vi "checkStatesBallPlacementEnemyTactic.vi"(9 "ballPosition(x,y)":dbl[](array[numeric]), 10 "Robot":refnum<class "Robot.lvclass">, 11 "Game in":refnum<class "Game.lvclass">) -> (1 "projectionOfQInBallPlacementLine":dbl[](array[numeric]) format="%#_13g", 2 "distance":dbl, 3 "isRobotIntereringInBallPlacement?":bool)   [LabVIEW 2021, in "BallPlacementEnemyTactic.lvclass"]
uses:
  BallPlacementEnemyTactic.lvclass
  Robot_class/Robot.lvclass
  D:/RoboIme/horie/SSL_AI/Object_class/Object.lvclass
  Game_class/Game.lvclass
  Object_class/Object.lvclass/Object.ctl
  Game_class/Game.lvclass/Game.ctl
  <vilib>/Analysis/baseanly.llb/Unit Vector (DBL).vi
  Game_class/Read Referee.vi
  Game_class/Read BallRef.vi
  Game_class/Read NewParameters.vi
  Object_class/Read x.vi
  Object_class/Read y.vi
  Referee_class/Referee.lvclass
  Ball_class/Ball.lvclass
  Utilities_class/Utilities.lvclass
  <vilib>/Analysis/NI_AALBase.lvlib
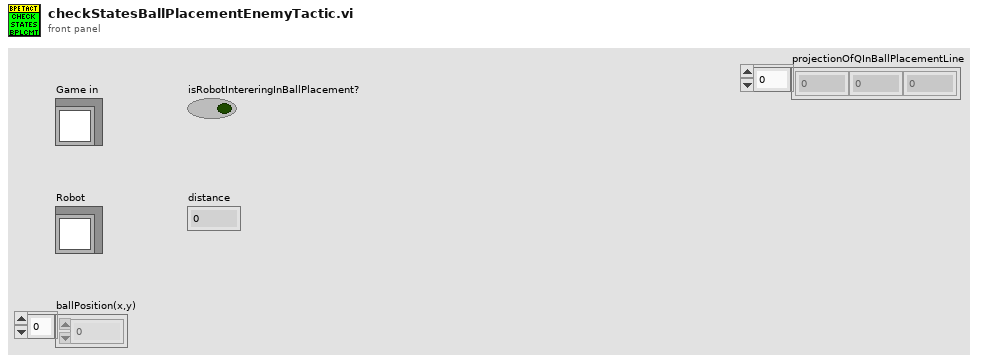
[diagram p1: front panel]
types:
  T1 = typedef "NewParameters.ctl" = cluster{"PenaltyDistance":dbl, "DistanceAttackerToBackBall":dbl, "Division":enum16{"Div B", "Div A"}, "DistanceToAvoidyEnemyRobot":dbl, "BallPlacementDistance":dbl, "DisatanceBehindBallToStealBall":dbl, "MaxDistanceToPositionKickoff":dbl, "BlockEnemyTarget":bool, "MaxStopVAng":dbl, "DistanceMarkerToEnemy":dbl, "IgnoreDribblerContact":bool, "DistanceToBeginEnemyPosession":dbl, "GoToBallWhenEnemyNotMoving":bool, "EnemyDistanceToReduceVelocity":dbl, "TurnOnEnemyDistanceToReduceVelocity":bool, "EnemyDistanceToShootOutBall":dbl, "DefenseKickBall":bool, "MoreKickToGoal? (0-0.3)":dbl, "ChipKickInEnemyField":bool, "ShootOutRobotId":dbl, "FieldLenghtDenominatorInShootOut":dbl, "AdjustPositionInBallPlacement":bool, "PowerGodPass":dbl, "VelocityAbortEnemyPos":dbl, "MaxDistToBeginPass":dbl, "MinDistToBeginPass":dbl, "VelocityInDirects":dbl, "BadDribblerIDs":i32[], "NewKickToDistanceAroundBall":dbl, "PowerAvoidColisionMarker":dbl, "DistanceToAvoidColisionMarker":dbl, "AvoidBallKick":dbl, "DistanceTryKick":dbl, "SuicideKickDIstance":dbl, "FirstKickAtck":bool, "AdjustFirstKickDistance":dbl, "FirstKickDefense":bool, "AvoidAimLessKick":dbl, "DistanceToAvoidyEnemyShootRobot ":dbl, "NumberOfMarkers":dbl, "PotField":bool, "PIDLateral":bool, "MinDistanceFirstKickX":dbl, "MinDistanceFirstKickY":dbl, "FractionOfDistToTouchGround\nAfterChipKick":dbl, "FractionOfKickxWhen\nComposedWithKickz":dbl, "Style":T2, "MoveInTurnState":bool, "DistFromEnemyToConsider\nMoveInTurnState":dbl, "CascadePID":bool, "TurnAroundParameters":cluster{"Radius":dbl, "Multiplier":dbl, "ChordAngle":dbl}, "SafeDriveVel":dbl, "DistanceToGoToBackBall":dbl, "minDistanceToNotFinishEnemyPossession":dbl, "TheBestKickers":i32[]}
  T2 = typedef "Style.ctl" = enum16{"Insanity", "Offensive", "Defensive"}
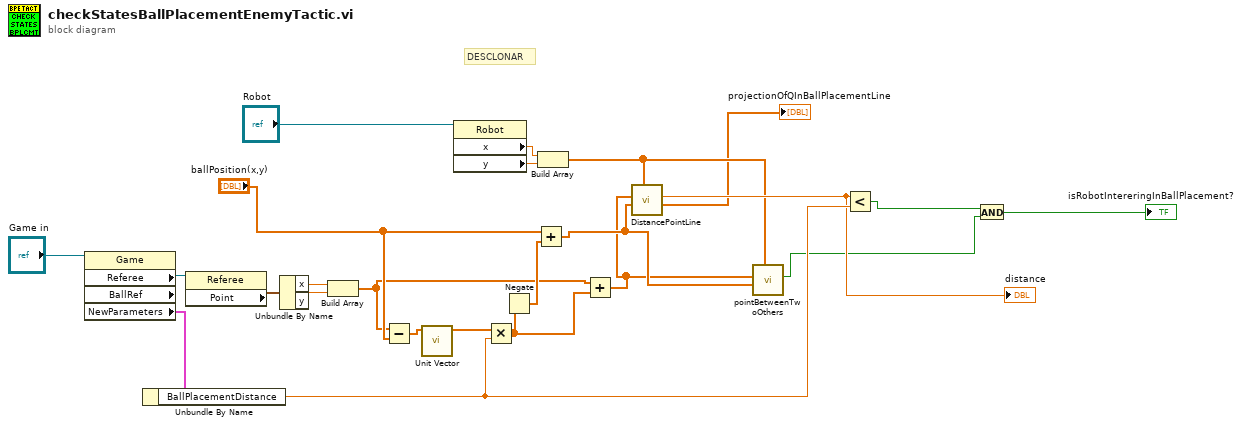
[diagram p0: block diagram]
diagram:
  # "DESCLONAR"
  n1 = property class="Game" props=["Referee", "BallRef", "NewParameters"](reference="Game in") -> ("Referee"=w3:refnum<class "Referee.lvclass">, "NewParameters"=w23:T1)  [unwired: 1 in, 3 out]
  n2 = Unbundle By Name(w23) -> ("BallPlacementDistance"=w24:dbl)
  n3 = property class="Referee"(reference=w3) -> ("Point"=w4:cluster{"x":sgl, "y":sgl})  [unwired: 1 in, 2 out]
  n4 = Unbundle By Name(w4) -> ("x"=w5:sgl, "y"=w6:sgl)
  n5 = Build Array(w5, w6) -> (w16:sgl[])
  n6 = Subtract(x=w16, y="ballPosition(x,y)") -> (x-y=w14:dbl[])
  n7 = call-poly <vilib>:"Unit Vector.vi"("Input Vector"=w14) -> ("Unit Vector"=w15:dbl[])  [unwired: 8 in, 2 out]
  n8 = property class="Robot"(reference="Robot") -> ("x"=w7:dbl, "y"=w8:dbl)  [unwired: 1 in, 2 out]
  n9 = Multiply(x=w15, y=w24) -> (x*y=w17:dbl[])
  n10 = Negate(x=w17) -> (-x=w19:dbl[])
  n11 = Add(x="ballPosition(x,y)", y=w19) -> (x+y=w20:dbl[])
  n12 = Build Array(w7, w8) -> (w12:dbl[])
  n13 = Add(x=w16, y=w17) -> (x+y=w18:dbl[])
  n14 = call "DistancePointLine.vi"("Q"=w12, "P2"=w20, "P1"=w18) -> ("projectionOfQInLineP1P2"=→"projectionOfQInBallPlacementLine":dbl[], "distance"=w21:dbl)  [unwired: 5 in, 2 out]
  "distance" <- w21
  n15 = call "pointBetweenTwoOthers.vi"("Query"=w12, "P2"=w20, "P1"=w18) -> ("queryBetweenP1P2"=w13:bool)  [unwired: 6 in, 2 out]
  n16 = Less?(x=w21, y=w24) -> (x < y?=w10:bool)
  n17 = And(x=w10, y=w13) -> (x .and. y?=→"isRobotIntereringInBallPlacement?":bool)
